vi "Full Table Handler.vi"(0 "Init":bool, 2 "DataTableRef":refnum<vi>, 3 "StatTableRef":refnum<vi>, 5 "table.Data":string[][](array[string]), 7 "table.Stats":string[][](array[string]), 9 "Data Row Index":i32=-999, 11 "Stat Row Index":i32=-999) -> ()   [LabVIEW 2019]
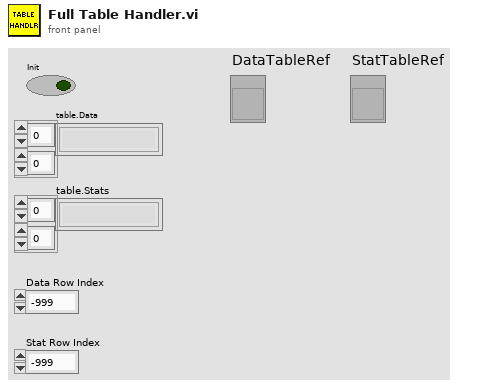
[diagram p1: front panel]
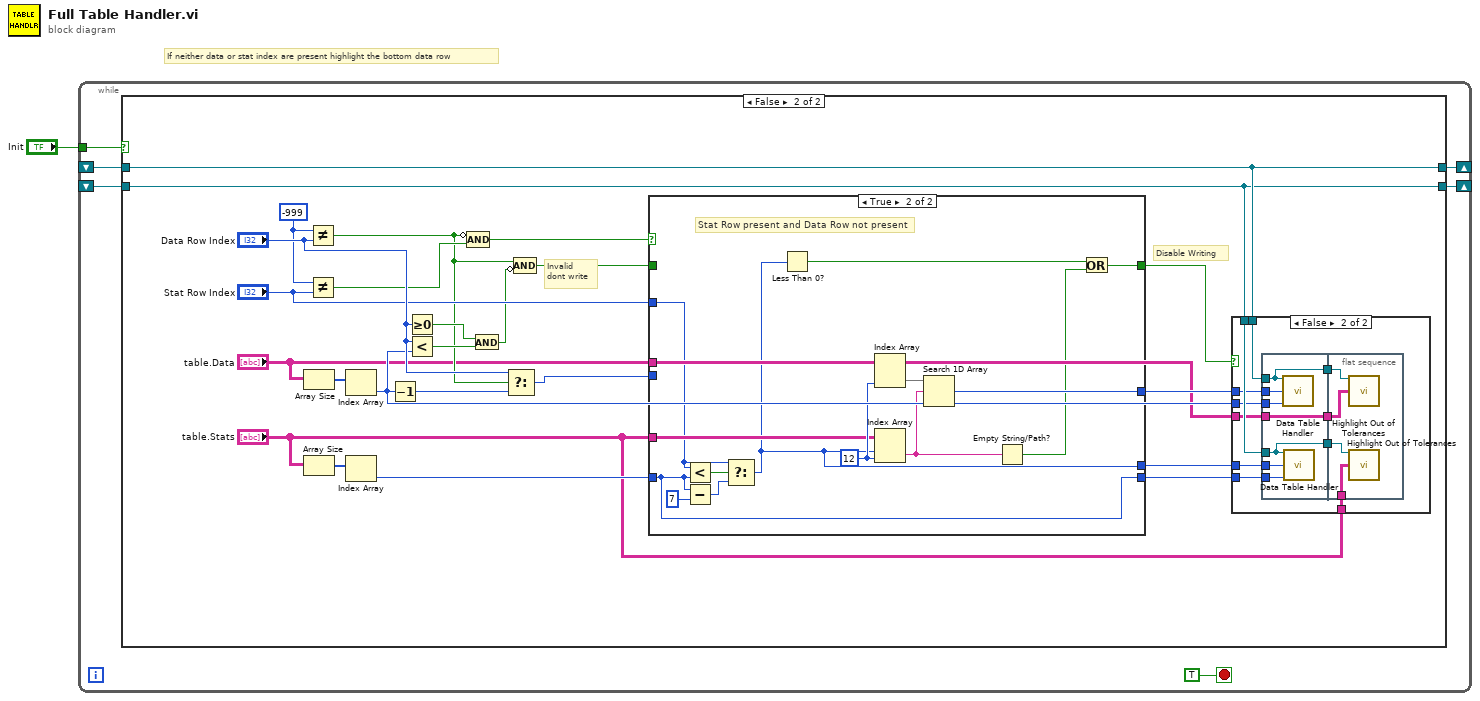
[diagram p0: block diagram]
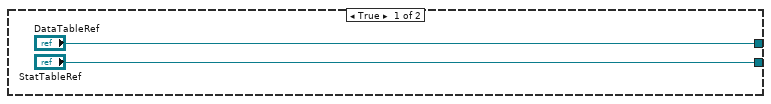
[diagram p2: hidden frame]
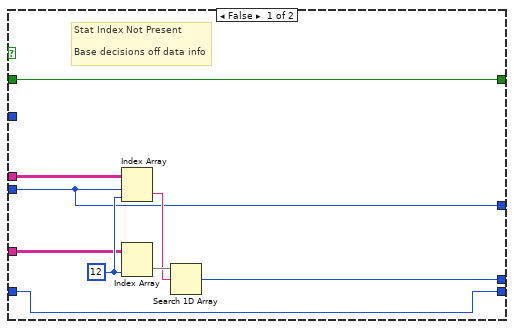
[diagram p4: hidden frame]
diagram:
  # "If neither data or stat index are present highlight the bottom data row"
  n1 = while {
    tunnel: "Init" -> [w6]
    shift-right: [w5] -> _
    shift-left: _ -> [w2]
    shift-right: [w4] -> _
    shift-left: _ -> [w3]
    stop <- TRUE stop-if-true
    n2 = case shown="False" w6 {
      tunnel: ["DataTableRef" w33] -> w5
      tunnel: ["StatTableRef" w32] -> w4
      tunnel: w3 -> [_ w32]
      tunnel: w2 -> [_ w33]
      frame True {
      }
      frame False {
        w24 = -999
        # "Disable Writing"
        # "Invalid\ndont write"
        n3 = Array Size(array="table.Data") -> (size(s)=w26:i32[])
        n4 = Array Size(array="table.Stats") -> (size(s)=w25:i32[])
        n5 = Not Equal?(x=w24, y="Data Row Index") -> (x != y?=w17:bool)
        n6 = Not Equal?(x=w24, y="Stat Row Index") -> (x != y?=w28:bool)
        n7 = Index Array(array=w26) -> (element=w21:i32)  [unwired: 1 in]
        n8 = Index Array(array=w25) -> (element=w13:i32)  [unwired: 1 in]
        n9 = Decrement(x=w21) -> (x-1=w27:i32)
        n10 = Greater Or Equal To 0?(x="Data Row Index") -> (x >= 0?=w18:bool)
        n11 = Less?(x="Data Row Index", y=w21) -> (x < y?=w19:bool)
        n12 = Compound Arithmetic op=AND(invert w17, w28) -> (w22:bool)
        n13 = And(x=w18, y=w19) -> (x .and. y?=w16:bool)
        n14 = Select(t="Data Row Index", s=w17, f=w27) -> (s? t:f=w20:i32)
        n15 = Compound Arithmetic op=AND(w17, invert w16) -> (w15:bool)
        n16 = case shown="True" w22 {
          tunnel: "table.Data" -> [w61 w78]
          tunnel: "table.Stats" -> [w60 w77]
          tunnel: w20 -> [w58 _]
          tunnel: [w59 w70] -> w30
          tunnel: [w58 w75] -> w31
          tunnel: "Stat Row Index" -> [_ w71]
          tunnel: [w57 w65] -> w14
          tunnel: w15 -> [w57 _]
          tunnel: w13 -> [w56 w69]
          tunnel: [w56 w69] -> w12
          frame False {
            w64 = 12 ("disabled index (col)")
            # "Stat Index Not Present\n\nBase decisions off data info"
            n17 = Index Array(array=w61, index (row)=w58, index (col)=w64) -> (element=w62:string)
            n18 = Index Array(array=w60, index (col)=w64) -> (element=w63:string[])  [unwired: 1 in]
            n19 = Search 1D Array(1D array=w63, element=w62) -> (index of element=w59:i32)  [unwired: 1 in]
          }
          frame True {
            w79 = 12 ("disabled index (col)")
            # "Stat Row present and Data Row not present"
            n20 = Less?(x=w71, y=w69) -> (x < y?=w74:bool)
            n21 = Subtract(x=w69, y=7) -> (x-y=w72:i32)
            n22 = Select(t=w71, s=w74, f=w72) -> (s? t:f=w70:i32)
            n23 = Less Than 0?(x=w70) -> (x < 0?=w66:bool)
            n24 = Index Array(array=w78, index (col)=w79) -> (element=w76:string[])  [unwired: 1 in]
            n25 = Index Array(array=w77, index (row)=w70, index (col)=w79) -> (element=w68:string)
            n26 = Search 1D Array(1D array=w76, element=w68) -> (index of element=w75:i32)  [unwired: 1 in]
            n27 = Empty String/Path?(string/path=w68) -> (empty?=w67:bool)
            n28 = Or(x=w66, y=w67) -> (x .or. y?=w65:bool)
          }
        }
        n29 = case shown="False" w14 {
          tunnel: w33 -> [_ w44]
          tunnel: w32 -> [_ w43]
          tunnel: w31 -> [_ w42]
          tunnel: w30 -> [_ w41]
          tunnel: w21 -> [_ w40]
          tunnel: w12 -> [_ w39]
          tunnel: "table.Data" -> [_ w37]
          tunnel: "table.Stats" -> [_ w36]
          frame True {
          }
          frame False {
            n30 = flat-sequence {
              tunnel: w44 -> [w46]
              tunnel: w43 -> [w45]
              tunnel: w42 -> [w51]
              tunnel: w41 -> [w50]
              tunnel: w40 -> [w49]
              tunnel: w39 -> [w48]
              tunnel: [w47] -> w38
              tunnel: w37 -> [w47]
              tunnel: [w46] -> w35
              tunnel: [w45] -> w34
              tunnel: w38 -> [w55]
              tunnel: w36 -> [w54]
              tunnel: w35 -> [w53]
              tunnel: w34 -> [w52]
              frame #0 {
                n31 = call "Data Table Handler.vi"("TableRef"=w46, "DesiredRow"=w51, "TableRows"=w49) -> ()  [unwired: 12 in, 1 out]
                n32 = call "Data Table Handler.vi"("TableRef"=w45, "DesiredRow"=w50, "TableRows"=w48) -> ()  [unwired: 12 in, 1 out]
              }
              frame #1 {
                n33 = call "Highlight Out of Tolerances.vi"("TableRef"=w53, "Array"=w55) -> ()  [unwired: 14 in]
                n34 = call "Highlight Out of Tolerances.vi"("TableRef"=w52, "Array"=w54) -> ()  [unwired: 14 in]
              }
            }
          }
        }
      }
    }
  }
